vi "Correct Error codes.vi"() -> ()   [LabVIEW 2017]
uses:
  String Subset.vi
  Parsing/Parse Full Path or Item Name.vi
  Offset/Find Item Locations by Path.vi
  JSONtext.lvlib
  <vilib>/addons/_JKI Toolkits/Caraya/classes/Test/Test.lvclass
  <vilib>/addons/_JKI Toolkits/Caraya/classes/Assert/Assert.lvclass
panel:
  out "Array 6":errorcluster[](array[cluster])
  out "Array 5":string[](array[string])
  out "Array 4":i32[](array[numeric])
  out "Array":bool[](array[boolean])
  out "Array 3":i32[](array[numeric])
  out "error out":errorcluster
  out "Array 2":errorcluster[](array[cluster])
  out "codes":i32[](array[numeric])
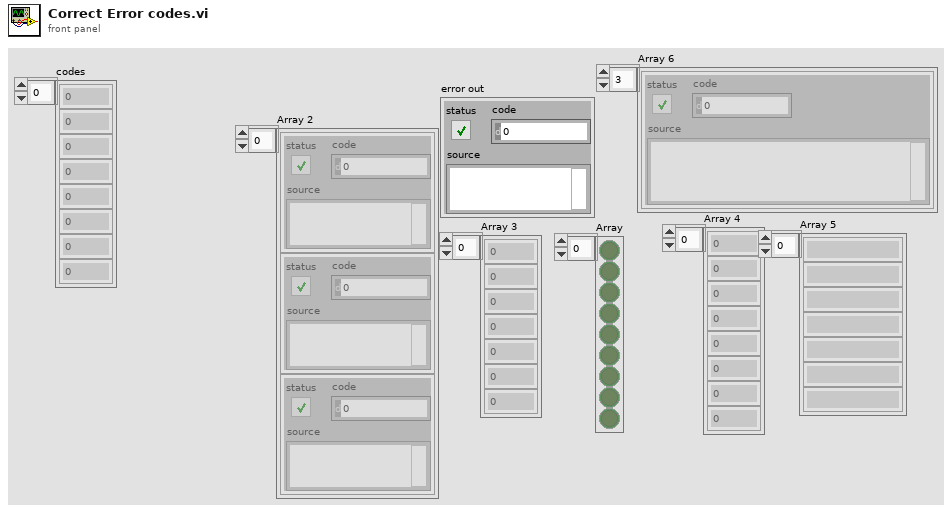
[diagram p1: front panel]
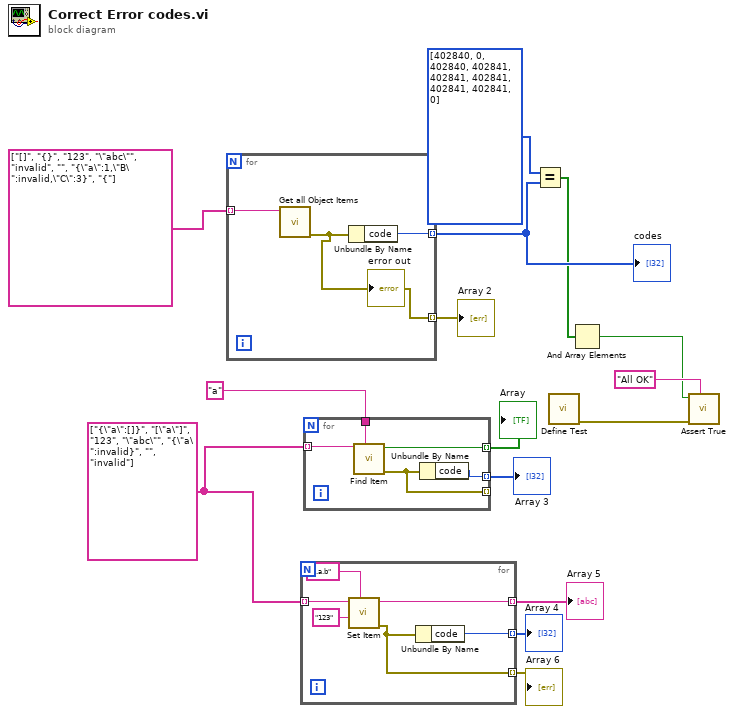
[diagram p0: block diagram]
diagram:
  w4 = string[] ["{\"a\":[]}", "[\"a\"]", "123", "\"abc\"", "{\"a\":invalid}", "", "invalid"] ("JSON")
  n1 = for {
    tunnel: string[] ["[]", "{}", "123", "\"abc\"", "invalid", "", "{\"a\":1,\"B\":invalid,\"C\":3}", "{"] ("JSON") -> [w17] mode=indexing
    tunnel: [w18] -> w14 mode=indexing
    tunnel: [w16] -> w7 mode=indexing
    n2 = call "Get all Object Items.vi"("JSON"=w17) -> ("error out"=w16:errorcluster)  [unwired: 7 in, 3 out]
    "error out" <- w16
    n3 = Unbundle By Name(w16) -> ("code"=w18:i32)
  }
  "codes" <- w14
  "Array 2" <- w7
  n4 = for {
    tunnel: w4 -> [w24] mode=indexing
    tunnel: [w21] -> w3 mode=indexing
    tunnel: [w20] -> w2 mode=indexing
    tunnel: [w19] -> w1 mode=indexing
    n5 = call "Set Item.vi"("$Path or Item Name"="$.a.b", "JSON to Insert"="123", "JSON"=w24) -> ("error out"=w19:errorcluster, "<JSON>"=w20:string)  [unwired: 5 in, 1 out]
    n6 = Unbundle By Name(w19) -> ("code"=w21:i32)
  }
  "Array 4" <- w3
  "Array 5" <- w2
  "Array 6" <- w1
  n7 = for {
    tunnel: w4 -> [w29] mode=indexing
    tunnel: "a" ("$Path or Item Name") -> [w28]
    tunnel: [w27] -> w6 mode=indexing
    tunnel: [w26] -> _ mode=indexing
    tunnel: [w25] -> w5 mode=indexing
    n8 = call "Find Item.vi"("$Path or Item Name"=w28, "JSON"=w29) -> ("error out"=w26:errorcluster, "Found"=w25:bool)  [unwired: 6 in, 2 out]
    n9 = Unbundle By Name(w26) -> ("code"=w27:i32)
  }
  "Array 3" <- w6
  "Array" <- w5
  n10 = Equal?(x=i32[] [402840, 0, 402840, 402841, 402841, 402841, 402841, 402841, 0] ("codes 2"), y=w14) -> (x = y?=w11:bool[])
  n11 = call <vilib>:"Define Test.vi"() -> ("error out"=w12:errorcluster)  [unwired: 11 in]
  n12 = And Array Elements(Boolean array=w11) -> (logical AND=w10:bool)
  n13 = call <vilib>:"Assert True.vi"("Label"="All OK", "error in (no error)"=w12, "True?"=w10) -> ()  [unwired: 8 in, 1 out]
